vi "SubConfocal_SetDiskSpinningSpeed.vi"(7 "Confocal scanner":T1={"SDC shutter"=FALSE, "Filter wheel"=6, "FW speed"=3, "Disk spinning"=FALSE, "Disk speed (rpm)"=3000.0} {"Disk speed (rpm)" min=1500.0 max=10000.0; "FW speed" min=1 max=5 step=1; "Filter wheel" items=["CFP"=1, "GFP"=2, "mCherry"=3, "Alexa-647"=4, "OFP"=5, "empty"=6]}, 8 "Error In":errorcluster, 11 "Confocal line (VISA IN)":refnum<visa-resource-name>="COM1") -> (0 "Error out":errorcluster, 3 "VISA OUT":refnum<visa-resource-name>)   [LabVIEW 2015]
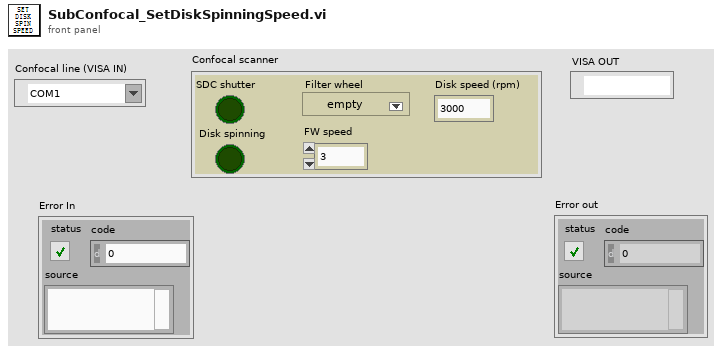
[diagram p1: front panel]
types:
  T1 = cluster{"SDC shutter":bool, "Filter wheel":u16, "FW speed":i32, "Disk spinning":bool, "Disk speed (rpm)":dbl}
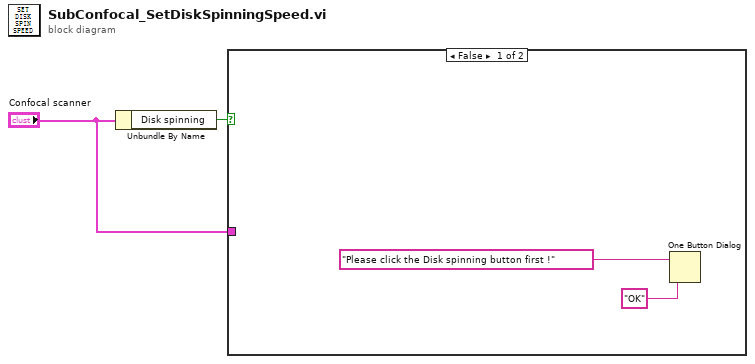
[diagram p0: block diagram]
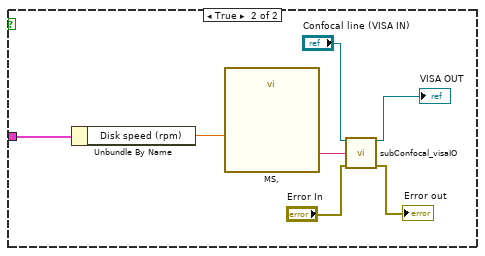
[diagram p2: hidden frame]
diagram:
  n1 = Unbundle By Name("Confocal scanner") -> ("Disk spinning"=w2:bool)
  n2 = case shown="False" w2 {
    tunnel: "Confocal scanner" -> [_ w5]
    frame False {
      n3 = One Button Dialog(message="Please click the Disk spinning button first !", button name ("OK")="OK") -> ()  [unwired: 1 out]
    }
    frame True {
      n4 = Unbundle By Name(w5) -> ("Disk speed (rpm)"=w6:dbl)
      n5 = call "MS,"("R"=w6) -> ("Result"=w11:string)  [unwired: 13 in, 1 out]
      n6 = call "subConfocal_visaIO.vi"("VISA  IN"="Confocal line (VISA IN)", "Command (to ctlr)"=w11, "error in"="Error In") -> ("VISA OUT"=→"VISA OUT":refnum<visa-resource-name>, "error out"=→"Error out":errorcluster)  [unwired: 8 in, 3 out]
    }
  }
